vi "开口率测试.vi"() -> ()   [LabVIEW 2011]
panel:
  in  "单一电压延时（ms）":u32=1000
  in  "循环次数":u32=10
  in  "循环测试":bool=TRUE
  in  "变化电压延时（ms）":u32=100
  in  "步进电压(V)":dbl=1.0
  in  "最小电压(V)":dbl
  in  "最大电压(V)":dbl=30.0
  in  "VISA资源名称":refnum<visa-resource-name>="GPIB0::1::INSTR"
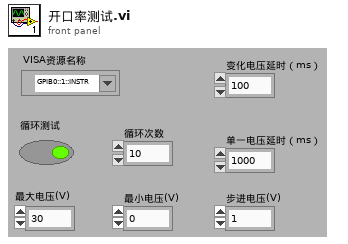
[diagram p1: front panel]
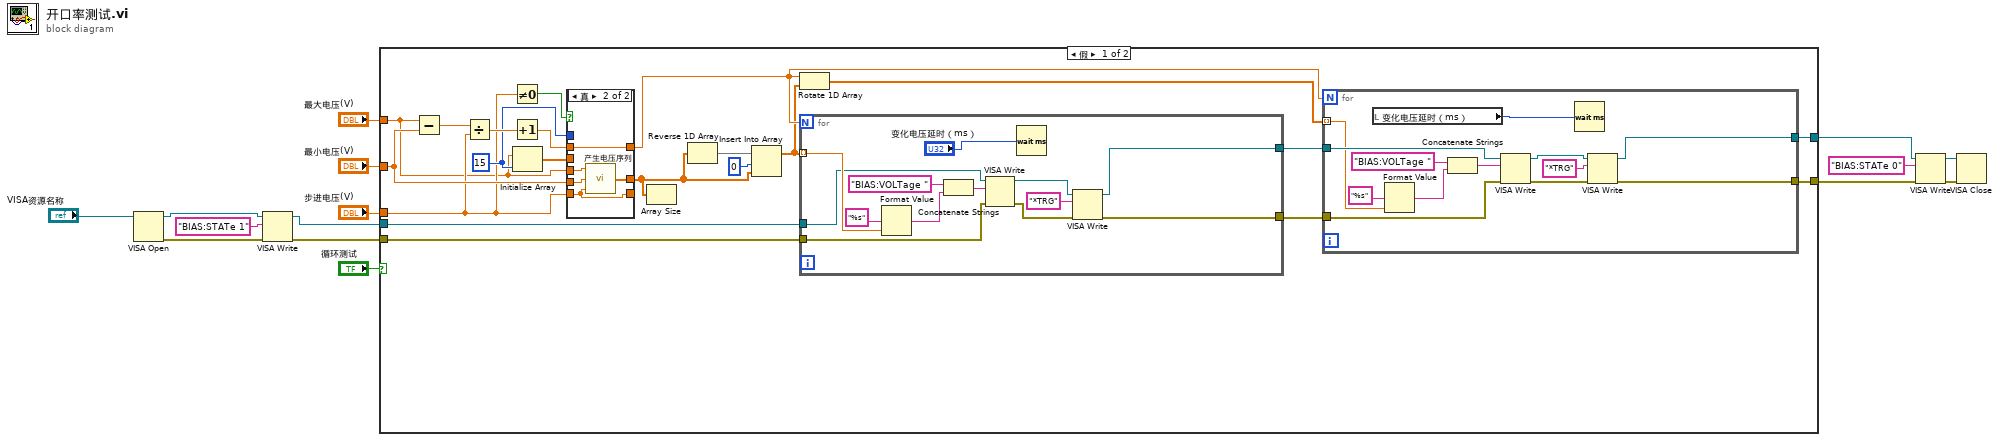
[diagram p0: block diagram]
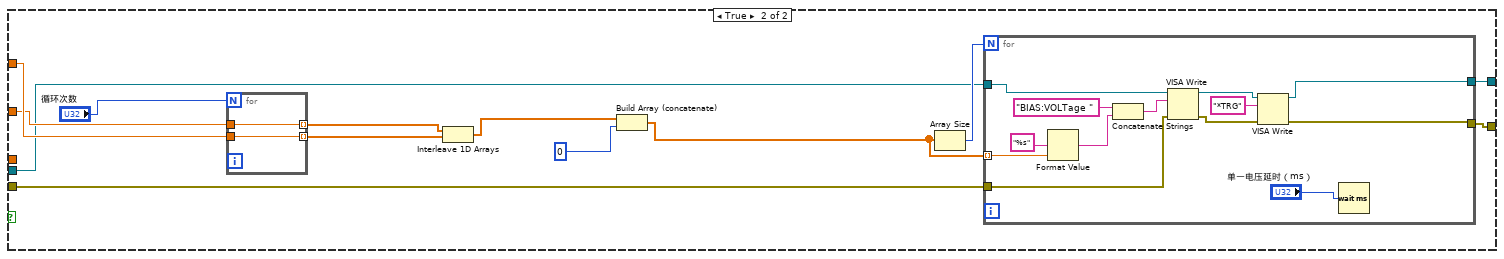
[diagram p3: hidden frame]
diagram:
  n1 = VISA Open(VISA resource name="VISA资源名称") -> (VISA resource name=w15:refnum<visa-resource-name>, error out=w12:errorcluster)  [unwired: 4 in]
  n2 = VISA Write(VISA resource name=w15, write buffer="BIAS:STATe 1" ("写入缓冲区"), error in (no error)=w12) -> (VISA resource name out=w4:refnum<visa-resource-name>, error out=w3:errorcluster)  [unwired: 1 out]
  n3 = case shown="假" "循环测试" {
    tunnel: "最小电压(V)" -> [w27 w82]
    tunnel: "步进电压(V)" -> [w26 _]
    tunnel: "最大电压(V)" -> [w25 w83]
    tunnel: w4 -> [w18 w79]
    tunnel: w3 -> [w19 w78]
    tunnel: [w17 w77] -> w2
    tunnel: [w16 w76] -> w1
    frame False {
      w30 = 15 ("维数大小")
      n4 = Subtract(x=w25, y=w27) -> (x-y=w36:dbl)
      n5 = Divide(x=w36, y=w26) -> (x/y=w35:dbl)
      n6 = Not Equal To 0?(x=w26) -> (x != 0?=w29:bool)
      n7 = Increment(x=w35) -> (x+1=w32:dbl)
      n8 = Initialize Array(w25, w30) -> (w31:dbl[])
      n9 = case shown="真" w29 {
        tunnel: w27 -> [_ w70]
        tunnel: w25 -> [_ w69]
        tunnel: w26 -> [w63 w66]
        tunnel: [w65 w68] -> w28
        tunnel: w32 -> [_ w67]
        tunnel: [w64 w67] -> w21
        tunnel: w31 -> [w65 _]
        tunnel: w30 -> [w64 _]
        tunnel: [w63 w66] -> _
        frame False {
        }
        frame True {
          n10 = call "产生电压序列.vi"("Delt"=w66, "Min"=w70, "Max"=w69) -> ("Array"=w68:dbl[])
        }
      }
      n11 = Array Size(array=w28) -> ()  [unwired: 1 out]
      n12 = Reverse 1D Array(array=w28) -> (reversed array=w33:dbl[])
      n13 = Insert Into Array(array=w33, index=0 ("索引"), new element=w28) -> (w20:dbl[])
      n14 = Rotate 1D Array(1:w20, 2:w21) -> (0:w24:dbl[])
      n15 = for {
        N: w21 -> [_]
        tunnel: [w51] -> w23
        tunnel: [w50] -> w22
        tunnel: w20 -> [w54] mode=indexing
        tunnel: w19 -> [w53]
        tunnel: w18 -> [w52]
        n16 = Format Value(format string="%s" ("格式字符串"), value (0)=w54) -> (output string=w58:string)  [unwired: 1 in]
        n17 = Concatenate Strings("BIAS:VOLTage " ("字符串"), w58) -> (w57:string)
        n18 = VISA Write(VISA resource name=w52, write buffer=w57, error in (no error)=w53) -> (VISA resource name out=w62:refnum<visa-resource-name>, error out=w61:errorcluster)  [unwired: 1 out]
        n19 = Wait (ms)(milliseconds to wait="变化电压延时（ms）") -> ()  [unwired: 1 out]
        n20 = VISA Write(VISA resource name=w62, write buffer="*TRG" ("写入缓冲区"), error in (no error)=w61) -> (VISA resource name out=w50:refnum<visa-resource-name>, error out=w51:errorcluster)  [unwired: 1 out]
      }
      n21 = for {
        N: w21 -> [_]
        tunnel: w22 -> [w49]
        tunnel: w23 -> [w48]
        tunnel: [w37] -> w16
        tunnel: [w38] -> w17
        tunnel: w24 -> [w39] mode=indexing
        n22 = local read "变化电压延时（ms）"() -> (w40:u32)
        n23 = Format Value(format string="%s" ("格式字符串"), value (0)=w39) -> (output string=w43:string)  [unwired: 1 in]
        n24 = Concatenate Strings("BIAS:VOLTage " ("字符串"), w43) -> (w42:string)
        n25 = VISA Write(VISA resource name=w49, write buffer=w42, error in (no error)=w48) -> (VISA resource name out=w47:refnum<visa-resource-name>, error out=w46:errorcluster)  [unwired: 1 out]
        n26 = Wait (ms)(milliseconds to wait=w40) -> ()  [unwired: 1 out]
        n27 = VISA Write(VISA resource name=w47, write buffer="*TRG" ("写入缓冲区"), error in (no error)=w46) -> (VISA resource name out=w38:refnum<visa-resource-name>, error out=w37:errorcluster)  [unwired: 1 out]
      }
    }
    frame True {
      n28 = for {
        N: "循环次数" -> [_]
        tunnel: w82 -> [w97]
        tunnel: w83 -> [w98]
        tunnel: [w98] -> w74 mode=indexing
        tunnel: [w97] -> w81 mode=indexing
      }
      n29 = Interleave 1D Arrays(w81, w74) -> (w73:dbl[])
      n30 = Build Array (concatenate)(w73, 0) -> (w71:dbl[])
      n31 = Array Size(array=w71) -> (size(s)=w80:i32)
      n32 = for {
        N: w80 -> [_]
        tunnel: [w84] -> w76
        tunnel: [w85] -> w77
        tunnel: w71 -> [w89] mode=indexing
        tunnel: w79 -> [w88]
        tunnel: w78 -> [w87]
        n33 = Format Value(format string="%s" ("格式字符串"), value (0)=w89) -> (output string=w92:string)  [unwired: 1 in]
        n34 = Concatenate Strings("BIAS:VOLTage " ("字符串"), w92) -> (w91:string)
        n35 = VISA Write(VISA resource name=w88, write buffer=w91, error in (no error)=w87) -> (VISA resource name out=w96:refnum<visa-resource-name>, error out=w95:errorcluster)  [unwired: 1 out]
        n36 = VISA Write(VISA resource name=w96, write buffer="*TRG" ("写入缓冲区"), error in (no error)=w95) -> (VISA resource name out=w85:refnum<visa-resource-name>, error out=w84:errorcluster)  [unwired: 1 out]
        n37 = Wait (ms)(milliseconds to wait="单一电压延时（ms）") -> ()  [unwired: 1 out]
      }
    }
  }
  n38 = VISA Write(VISA resource name=w2, write buffer="BIAS:STATe 0" ("写入缓冲区"), error in (no error)=w1) -> (VISA resource name out=w9:refnum<visa-resource-name>, error out=w10:errorcluster)  [unwired: 1 out]
  n39 = VISA Close(VISA resource name=w9, error in (no error)=w10) -> ()  [unwired: 1 out]
